vi "Niveles_tanques.vi"() -> ()   [LabVIEW 2020]
panel:
  in  "Niveles tanques":T1 {"Cera" scale=0.0..100.0; "Tanque de agua" scale=0.0..100.0; "Detergente" scale=0.0..100.0}
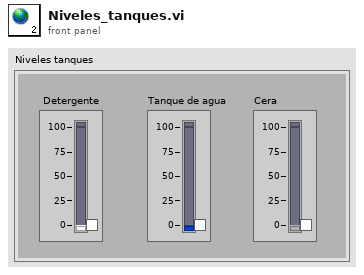
[diagram p1: front panel]
types:
  T1 = cluster{"Detergente":dbl, "Tanque de agua":dbl, "Cera":dbl}
diagram:
